vi "NanoStep GetParams.vi"(0 "VISA Rsrc":refnum<visa-resource-name>="GPIB1::15::INSTR", 5 "Axis":u16(ring)=1 items=["Axis 0", "Axis 1", "All Axis"], 11 "error in":errorcluster) -> (6 "Axis Parameters":T1={"Resolution\n(Stp/mm)"=0.5, "InitVelocity"=0.5, "MaxVelocity"=0.5, "Accel"=0.5, "Stage Type"=0} {"Stage Type" items=["Linear", "Rotary"]}, 15 "error out":errorcluster)   [LabVIEW 2010]
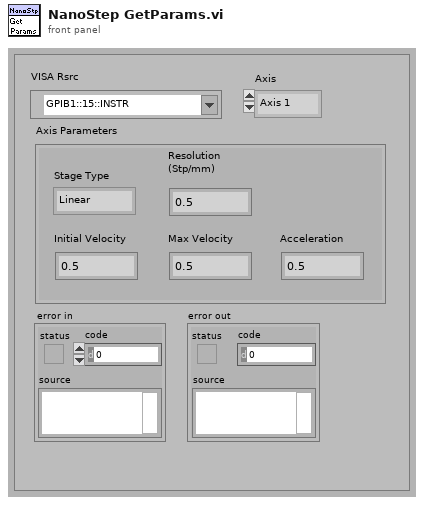
[diagram p1: front panel]
types:
  T1 = cluster{"Resolution\n(Stp/mm)":dbl, "InitVelocity":dbl, "MaxVelocity":dbl, "Accel":dbl, "Stage Type":u16}
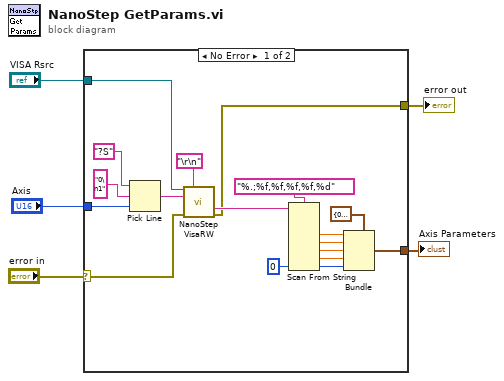
[diagram p0: block diagram]
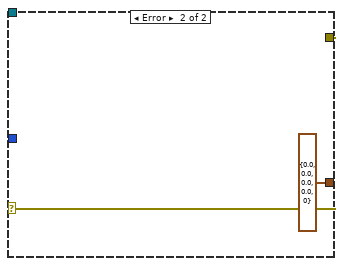
[diagram p2: hidden frame]
diagram:
  n1 = case shown="No Error" "error in" {
    selector: "error in" -> [w23 w25]
    tunnel: "Axis" -> [w20 _]
    tunnel: [w11 w25] -> w3
    tunnel: "VISA Rsrc" -> [w22 _]
    tunnel: [w10 T1 {"Resolution\n(Stp/mm)"=0.0, "InitVelocity"=0.0, "MaxVelocity"=0.0, "Accel"=0.0, "Stage Type"=0} ("Axis Parameters")] -> w1
    frame No Error {
      n2 = Pick Line(string ("")="?S" ("chaîne (\"\")"), multi-line string="0\n1" ("x"), line index=w20) -> (output string=w18:string)
      n3 = call <userlib>:"NanoStep VisaRW.vi"("VISA Rsrc"=w22, "EOS (Aucun)"="\r\n", "ChaineCom"=w18, "error in (no error)"=w23) -> ("ChaineRep"=w16:string, "error out"=w11:errorcluster)  [unwired: 8 in, 2 out]
      n4 = Scan From String(format string="%.;%f,%f,%f,%f,%d" ("chaîne de format"), input string=w16, default 5=u16 0 ("valeur par défaut 5")) -> (output 1=w9:dbl, output 2=w8:dbl, output 3=w7:dbl, output 4=w6:dbl, output 5=w13:u16)  [unwired: 6 in, 3 out]
      n5 = Bundle(cluster=T1 {"Resolution\n(Stp/mm)"=0.5, "InitVelocity"=0.5, "MaxVelocity"=0.5, "Accel"=0.5, "Stage Type"=1} ("Axis Parameters"), "Resolution\n(Stp/mm)"=w9, "InitVelocity"=w8, "MaxVelocity"=w7, "Accel"=w6, "Stage Type"=w13) -> (w10:T1)
    }
    frame Error {
    }
  }
  "error out" <- w3
  "Axis Parameters" <- w1
